vi "Pressure Monitor GUI.vi"(9 "Standalone":bool=TRUE, 10 "Init Data":variant, 11 "My Name":string) -> ()   [LabVIEW 2024]
uses:
  typedefs/CC enum Operation Mode.ctl
  Subsystems/SS typedef cluster Instrument Command Queue Data.ctl
  Subsystems/SS cluster Data Queue type.ctl
  hk-channel-class/hk-channel-class/HK Item/HK Item.lvclass
  CryoCooler/Cryo Cooler/CryoCoolerAVC/CryoCoolerAVC Command cluster.ctl
  CryoCooler/Cryo Cooler/CryoCoolerAVC/CryoCoolerAVC Command enum.ctl
  Pressure Monitor/Pressure Monitor.lvclass
  typedefs/CC cluster Alarm Data.ctl
  Pressure Monitor/CC cluster Pressure Monitor Settings.ctl
  Pressure Monitor/Lesker Pressure/Lesker Pressure.lvclass
  Pressure Monitor/MKS/MKS.lvclass
  hk-channel-class/hk-channel-class/HK Item/HK Item.lvclass/HK Item.ctl
  hk-channel-class/hk-channel-class/HK Item/HK Channel cluster Telemetry Data.ctl
  hk-channel-class/hk-channel-class/HK Item/HK Channel enum Data Type.ctl
  <vilib>/Utility/error.llb/DialogType.ctl
  Pressure Monitor/Lesker Pressure/Lesker Pressure.lvclass/Lesker Pressure.ctl
  hk-channel-class/hk-channel-class/HK Item/Write Source.vi
  CryoCooler/Cryo Cooler/CryoCoolerAVC/CryoCoolerAVC.lvclass
panel:
  in  "Mode":T1
  in  "Tab Control":enum32{"Pressure Monitor", "Engineering", "Log"}(tab)
  in  "Reconnect":bool
  in  "Clear History":bool
  in  "Log Scale":bool=TRUE
  out "Alarm Message":string
  out "Pressure Connected":bool
  out "Alarm":bool
  in  "Status":i32[](listbox) caption="Pressure Monitor"
  out "XY Graph":T2(graph)
  in  "Lesker Notes":string="Guage type is 392\nIf the Ion Gauge commands to turn the filament ON and OFF returns a SYNTAX Error, then you\nneed to go to the gauge front panel menu and select:\nFirst TURN IG OFF, then\nSETUP UNIT > IG CNTL > Set to RS485\n\nSee page 30 of the manual"
  in  "Inst Filament":bool caption="Filament"
  in  "Pump Filament":bool
  in  "Pressure Alarm Level":dbl format="%^_3g"
  in  "Enable Pump Reading?":bool
  in  "Pump Addr":refnum<visa-resource-name>
  in  "Instrument Addr":refnum<visa-resource-name>
  in  "Pressure Type":u16(ring) items=["Simulation", "Lesker", "MKS"]
  in  "Close":bool
  out "Log":string
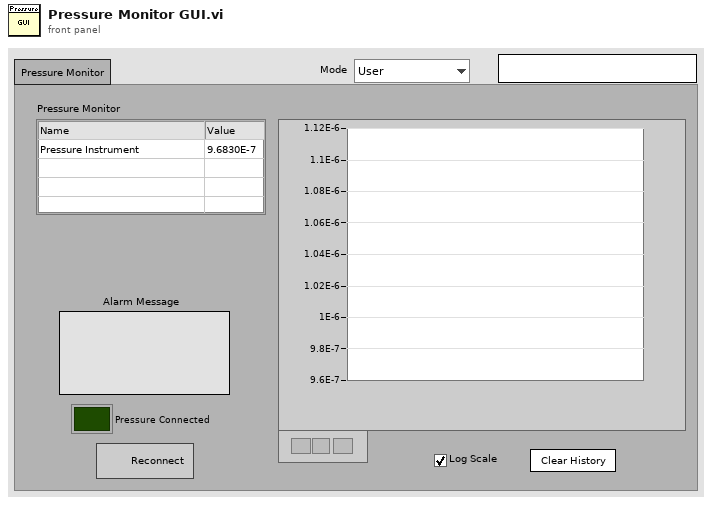
[diagram p1: front panel]
types:
  T1 = typedef "CC enum Operation Mode.ctl" = enum16{"User", "Engineering"}
  T2 = cluster{cluster{"Time Stamp":timestamp, "Numeric":dbl}[]}[]
  T3 = typedef "SS typedef cluster Instrument Command Queue Data.ctl" = cluster{"Cmd":string, "Parameters":variant}
  T4 = typedef "CryoCoolerAVC.lvclass/CryoCoolerAVC Command cluster.ctl" = cluster{"Command":T5, "Options":string, "Cryo Idx":i32}
  T5 = typedef "CryoCoolerAVC.lvclass/CryoCoolerAVC Command enum.ctl" = u16
  T6 = typedef "CC cluster Alarm Data.ctl" = cluster{"Measured Value":dbl, "Alarm Low":dbl, "Alarm High":dbl, "Message":string, "Source":string}
  T7 = typedef "CC cluster Pressure Monitor Settings.ctl" = cluster{"Lesker Addrs":refnum<visa-resource-name>[], "Enabled?":bool[], "Pressure Alarm Level":dbl, "Filaments":bool[]}
  T8 = cluster{"state":refnum<user-event>, "cmd q":refnum<queue>, "Cmd":T3, "Data Q":refnum<queue>, "error":errorcluster, "next poll":timestamp, "My Name":string, "poll":bool, "Channel List":refnum<class "HK Item.lvclass">[], "Focus Pos":dbl, "Data":dbl[], "Cryo Cmd":T4, "Alarm":bool, "PM Ref":refnum<class "Pressure Monitor.lvclass">, "Alarms":T6[], "Source":string, "Settings":T7}
  T9 = typedef "SS cluster Data Queue type.ctl" = cluster{"Source":string, "Type":string, "Data":variant}
  T10 = typedef "HK Item.lvclass/HK Channel enum Data Type.ctl" = enum16{"Floating Point", "Integer", "Enum", "String", "Waveform", "File"}
  T11 = typedef "HK Item.lvclass/HK Channel cluster Telemetry Data.ctl" = cluster{"Ch Names":string[], "Ch Values":dbl[], "Timestamp":timestamp, "Data Type":T10}
  T12 = typedef "CC cluster Device Index.ctl" = cluster{"Device Type Name":string, "Curr Device Name":string, "All Instances":string[]}
  T13 = cluster{"Select Ch":i32[], "Default Device":string}
  T14 = typedef "HK Item.lvclass/HK Channel Units and Setup.ctl" = cluster{"Unit Type":string, "Units":string, "Configuration":string, "Digits":i32, "Data Type":T10, "Exponential?":bool, "Source":string}
  T15 = cluster{cluster{"Time Stamp":timestamp, "Numeric":dbl}[]}
  T16 = typedef "DialogType.ctl" = u16
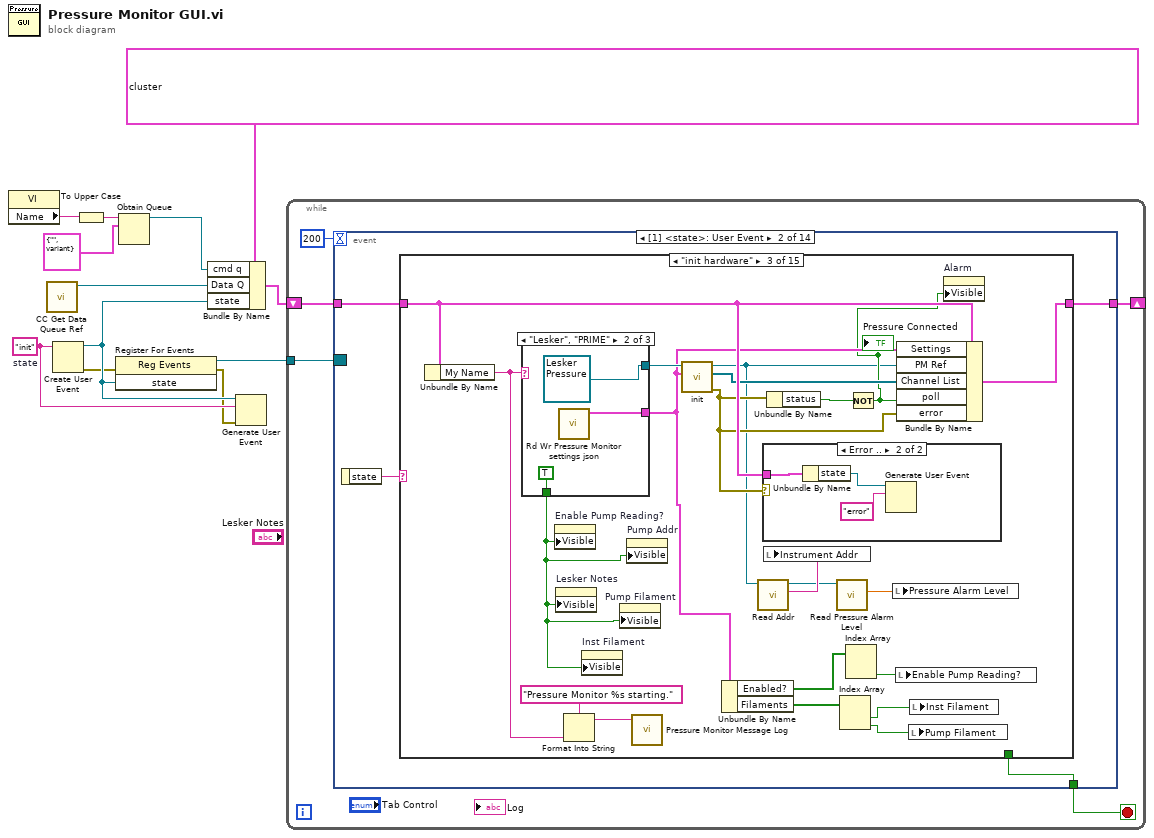
[diagram p0: block diagram]
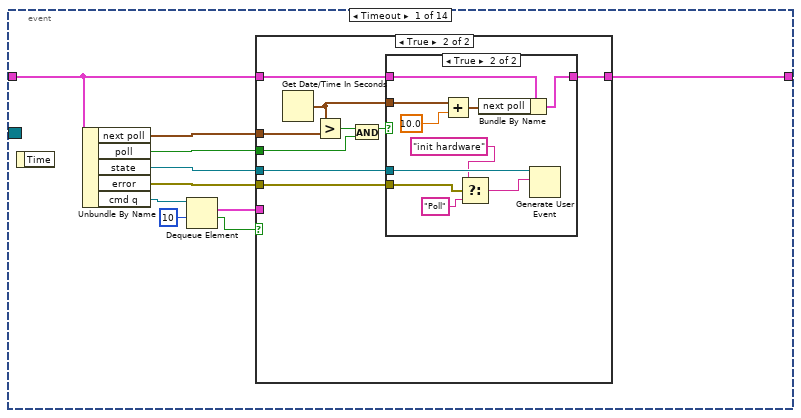
[diagram p2: hidden frame]
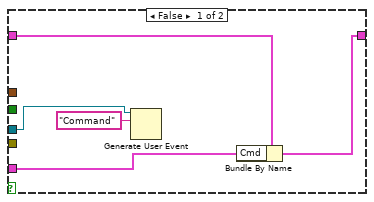
[diagram p3: hidden frame]
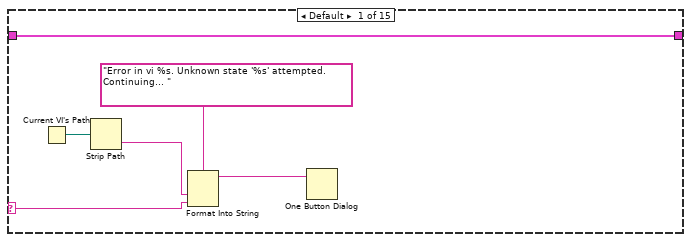
[diagram p5: hidden frame]
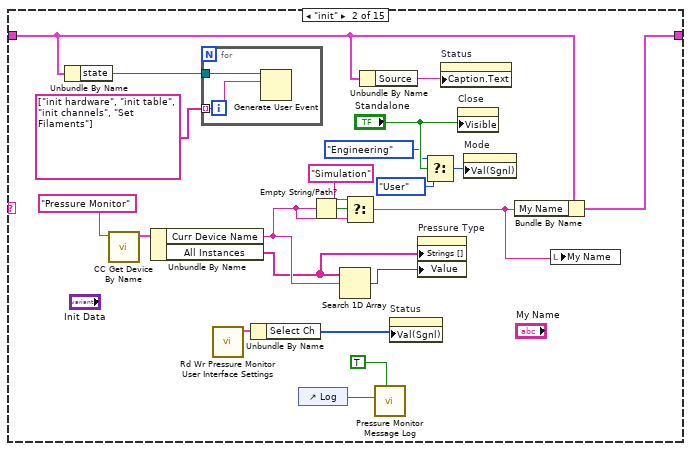
[diagram p6: hidden frame]
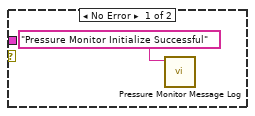
[diagram p7: hidden frame]
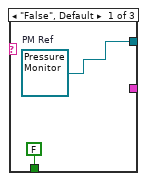
[diagram p8: hidden frame]
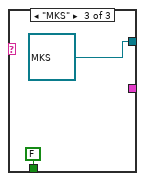
[diagram p9: hidden frame]
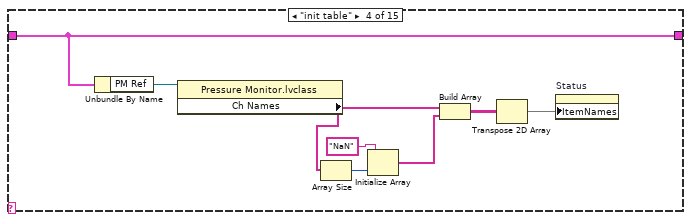
[diagram p10: hidden frame]
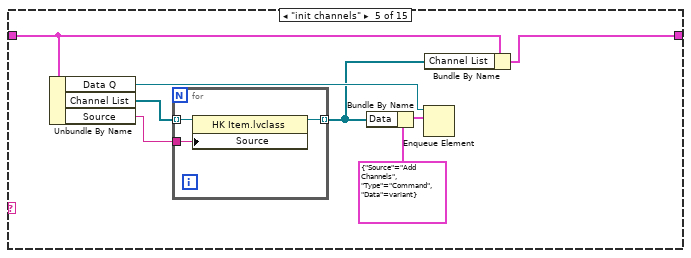
[diagram p11: hidden frame]
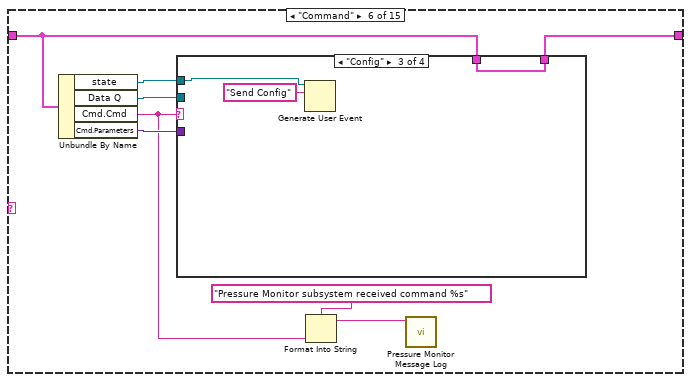
[diagram p12: hidden frame]
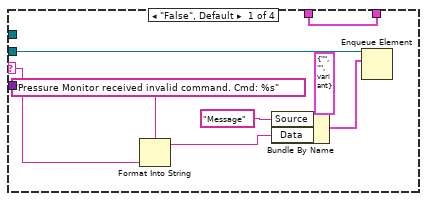
[diagram p13: hidden frame]
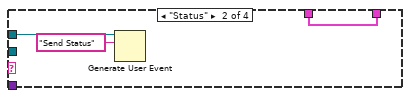
[diagram p14: hidden frame]
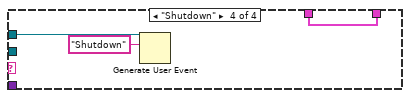
[diagram p15: hidden frame]
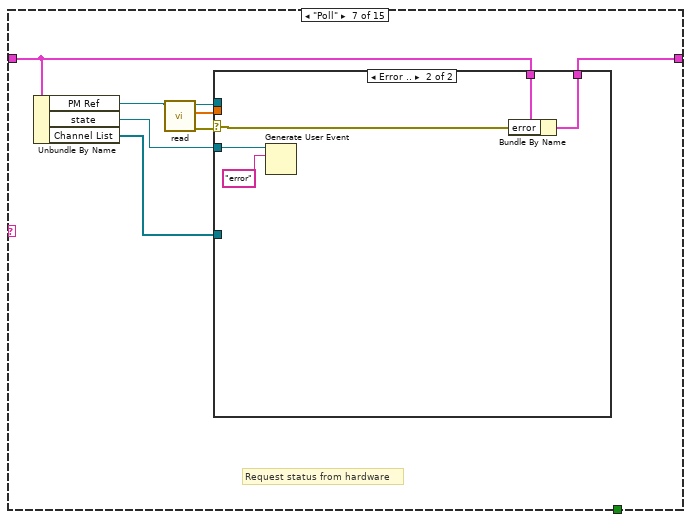
[diagram p16: hidden frame]
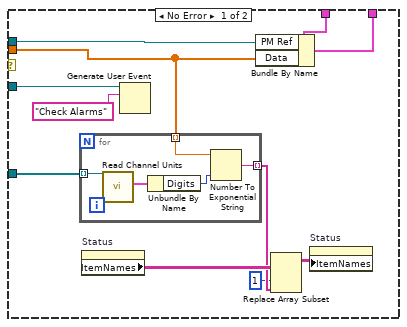
[diagram p17: hidden frame]
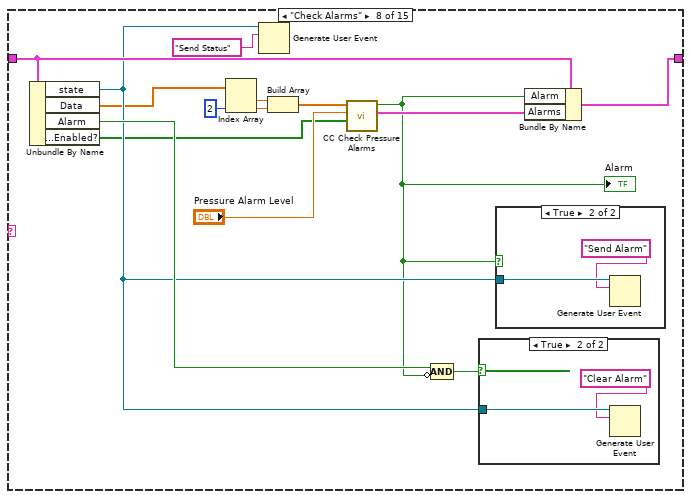
[diagram p18: hidden frame]
diagram:
  w8 = "init"  # state
  n1 = property class="VI"() -> ("Name"=w4:string)  [unwired: 2 in, 2 out]
  n2 = call "CC Get Data Queue Ref.vi"() -> ("Data Q"=w5:refnum<queue>)  [unwired: 10 in, 1 out]
  n3 = Create User Event(user event datatype=w8) -> (user event=w10:refnum<user-event>, error out=w6:errorcluster)  [unwired: 1 in]
  n4 = To Upper Case(1:w4) -> (0:w3:string)
  n5 = register-events(error in=w6, w10) -> (reference out=w9:refnum<event-registration>, error out=w7:errorcluster)  [unwired: 1 in]
  n6 = Obtain Queue(name (unnamed)=w3, element data type=T3 {"Cmd"="", "Parameters"=variant}) -> (queue out=w1:refnum<queue>)  [unwired: 3 in, 2 out]
  n7 = Bundle By Name(cluster=T8 {"state"=refnum, "cmd q"=refnum, "Cmd"={"Cmd"="", "Parameters"=variant}, "Data Q"=refnum, "error"={"status"=FALSE, "code"=0, "source"=""}, "next poll"=timestamp(0 s since 1904-01-01), "My Name"="", "poll"=FALSE, "Channel List"=[], "Focus Pos"=0.0, "Data"=[], "Cryo Cmd"={"Command"=0, "Options"="", "Cryo Idx"=0}, "Alarm"=FALSE, "PM Ref"=refnum, "Alarms"=[], "Source"="Pressure Monitor", "Settings"={"Lesker Addrs"=[], "Enabled?"=[], "Pressure Alarm Level"=0.0001, "Filaments"=[]}}, "cmd q"=w1, "Data Q"=w5, "state"=w10) -> (w11:T8)
  n8 = Generate User Event(user event=w10, event data cluster=w8, error in=w7) -> ()  [unwired: 1 in, 2 out]
  n9 = while {
    tunnel: w9 -> [w17]
    shift-right: [w15] -> _
    shift-left: w11 -> [w16]
    stop <- w14 stop-if-true
    n10 = event shown="[1] <state>: User Event" {
      selector: w17 -> [_ _ _ _ _ _ _ _ _ _ _ _ _ _]
      dyn-events: _ -> [_ _ _ _ _ _ _ _ _ _ _ _ _ _]
      timeout: 200 -> [_ _ _ _ _ _ _ _ _ _ _ _ _ _]
      tunnel: w16 -> [w22 w55 w297 w300 w307 w310 w315 w317 w345 w357 w371 w376 w382 w385]
      tunnel: [w21 w54 w297 w301 w307 w310 w315 w318 w345 w358 w371 w376 w382 w385] -> w15
      tunnel: [_ w53 _ _ _ _ _ _ _ _ _ _ _ _] -> w14
      event Timeout {
        n11 = event-data() -> ()  [unwired: 1 in, 1 out]
        n12 = Unbundle By Name(w22) -> ("next poll"=w20:timestamp, "poll"=w19:bool, "state"=w23:refnum<user-event>, "error"=w18:errorcluster, "cmd q"=w27:refnum<queue>)
        n13 = Dequeue Element(queue=w27, timeout in ms (-1)=10) -> (element=w24:T3, timed out?=w25:bool)  [unwired: 1 in, 2 out]
        n14 = case shown="True" w25 {
          tunnel: w24 -> [w29 _]
          tunnel: w23 -> [w32 w38]
          tunnel: w22 -> [w30 w39]
          tunnel: [w28 w36] -> w21
          tunnel: w20 -> [_ w41]
          tunnel: w19 -> [_ w34]
          tunnel: w18 -> [_ w33]
          frame False {
            n15 = Generate User Event(user event=w32, event data cluster="Command" ("event data")) -> ()  [unwired: 2 in, 2 out]
            n16 = Bundle By Name(cluster=w30, "Cmd"=w29) -> (w28:T8)
          }
          frame True {
            n17 = Get Date/Time In Seconds() -> (seconds since 1Jan1904=w37:timestamp)
            n18 = Greater?(x=w37, y=w41) -> (0:w40:bool)
            n19 = And(x=w40, y=w34) -> (x .and. y?=w35:bool)
            n20 = case shown="True" w35 {
              tunnel: w39 -> [w42 w52]
              tunnel: w38 -> [_ w51]
              tunnel: w37 -> [_ w50]
              tunnel: [w42 w47] -> w36
              tunnel: w33 -> [_ w45]
              frame False {
              }
              frame True {
                n21 = Add(x=w50, y=10.0) -> (x+y=w48:timestamp)
                n22 = Select(t="init hardware" ("event data"), s=w45, f="Poll" ("event data")) -> (s? t:f=w43:string)
                n23 = Bundle By Name(cluster=w52, "next poll"=w48) -> (w47:T8)
                n24 = Generate User Event(user event=w51, event data cluster=w43) -> ()  [unwired: 2 in, 2 out]
              }
            }
          }
        }
      }
      event User Event {
        n25 = event-data() -> ("state"=w56:string)  [unwired: 1 in]
        n26 = case shown="\"init hardware\"" w56 {
          selector: w56 -> [w61 _ _ _ _ _ _ _ _ _ _ _ _ _ _]
          tunnel: w55 -> [w57 w64 w103 w125 w126 w140 w168 w203 w222 w230 w247 w252 w263 w269 w293]
          tunnel: [w57 w82 w106 w125 w127 w141 w169 w204 w222 w230 w247 w253 w264 w270 w293] -> w54
          tunnel: [_ _ _ _ _ _ _ _ _ _ _ _ _ _ TRUE] -> w53
          frame Default {
            n27 = Current VI's Path() -> (path=w60:path)
            n28 = Strip Path(path=w60) -> (name=w59:string)  [unwired: 1 out]
            n29 = Format Into String(format string="Error in vi %s. Unknown state '%s' attempted. Continuing... ", w59, w61) -> (resulting string=w58:string)  [unwired: 2 in, 1 out]
            n30 = One Button Dialog(message=w58) -> ()  [unwired: 1 in, 1 out]
          }
          frame "init" {
            n31 = Unbundle By Name(w64) -> ("state"=w81:refnum<user-event>)
            n32 = call "CC Get Device By Name.vi"("Device Type"="Pressure Monitor") -> ("Device"=w76:T12)  [unwired: 8 in, 2 out]
            n33 = Unbundle By Name(w76) -> ("Curr Device Name"=w75:string, "All Instances"=w74:string[])
            n34 = for {
              tunnel: w81 -> [w85]
              tunnel: string[] ["init hardware", "init table", "init channels", "Set Filaments"] -> [w84] mode=indexing
              n35 = Generate User Event(user event=w85, event data cluster=w84) -> ()  [unwired: 2 in, 2 out]
            }
            n36 = call "Rd Wr Pressure Monitor User Interface Settings.vi"() -> ("Settings"=w66:T13)  [unwired: 10 in, 1 out]
            n37 = Unbundle By Name(w66) -> ("Select Ch"=w65:i32[])
            n38 = control-ref of="Log"() -> (w69:refnum<vi>)
            n39 = Empty String/Path?(string/path=w75) -> (empty?=w83:bool)
            n40 = Search 1D Array(1D array=w74, element=w75) -> (index of element=w79:i32)  [unwired: 1 in]
            n41 = Select(t="Simulation", s=w83, f=w75) -> (s? t:f=w67:string)
            n42 = Unbundle By Name(w64) -> ("Source"=w63:string)
            n43 = call "Pressure Monitor Message Log.vi"("init?"=TRUE, "Log Ref"=w69) -> ()  [unwired: 8 in, 2 out]
            n44 = property on="Status" class="MCListbox (strict)"("Val(Sgnl)"=w65) -> ()  [unwired: 2 in, 2 out]
            n45 = property on="Pressure Type" class="Ring (strict)"("Strings []"=w74, "Value"=w79) -> ()  [unwired: 2 in, 2 out]
            n46 = Select(t=CC_enum_Operation_Mode."Engineering" ("Mode"), s="Standalone", f=CC_enum_Operation_Mode."User" ("Mode")) -> (s? t:f=w70:T1)
            n47 = property on="Status" class="MCListbox (strict)"("Caption.Text"=w63) -> ()  [unwired: 2 in, 2 out]
            n48 = property on="Close" class="Bool"("Visible"="Standalone") -> ()  [unwired: 2 in, 2 out]
            n49 = property on="Mode" class="Enum (strict)"("Val(Sgnl)"=w70) -> ()  [unwired: 2 in, 2 out]
            n50 = Bundle By Name(cluster=w64, "My Name"=w67) -> (w82:T8)
            n51 = local write "My Name"(w67) -> ()
          }
          frame "init hardware" {
            n52 = Unbundle By Name(w103) -> ("My Name"=w105:string)
            n53 = case shown="\"Lesker\", \"PRIME\"" w105 {
              tunnel: [w112 refnum<class "Lesker Pressure.lvclass"> refnum ("Lesker Pressure.lvclass") refnum<class "MKS.lvclass"> refnum ("MKS.lvclass")] -> w101
              tunnel: [_ w115 _] -> w96
              tunnel: [FALSE TRUE FALSE] -> w90
              frame "False", Default {
                w112 = refnum<class "Pressure Monitor.lvclass"> refnum  # PM Ref
              }
              frame "Lesker", "PRIME" {
                n54 = call "Rd Wr Pressure Monitor settings json.vi"() -> ("Pressur Monitor Settings"=w115:T7)  [unwired: 10 in, 1 out]
              }
              frame "MKS" {
              }
            }
            n55 = property on="Enable Pump Reading?" class="Bool (strict)"("Visible"=w90) -> ()  [unwired: 2 in, 2 out]
            n56 = property on="Lesker Notes" class="Str"("Visible"=w90) -> ()  [unwired: 2 in, 2 out]
            n57 = Format Into String(format string="Pressure Monitor %s starting.", w105) -> (resulting string=w102:string)  [unwired: 2 in, 1 out]
            n58 = property on="Inst Filament" class="Bool (strict)"("Visible"=w90) -> ()  [unwired: 2 in, 2 out]
            n59 = property on="Pump Filament" class="Bool (strict)"("Visible"=w90) -> ()  [unwired: 2 in, 2 out]
            n60 = property on="Pump Addr" class="VISAName"("Visible"=w90) -> ()  [unwired: 2 in, 2 out]
            n61 = call "Pressure Monitor Message Log.vi"("String in"=w102) -> ()  [unwired: 9 in, 2 out]
            n62 = call-dynamic "init.vi"("Init Data"=w96, "Pressure Monitor in"=w101) -> ("error out"=w99:errorcluster, "Channel List"=w100:refnum<class "HK Item.lvclass">[], "Pressure Monitor out"=w89:refnum<class "Pressure Monitor.lvclass">)  [unwired: 7 in]
            n63 = Unbundle By Name(w96) -> ("Enabled?"=w98:bool[], "Filaments"=w95:bool[])
            n64 = call-dynamic "Read Addr.vi"("Pressure Monitor in"=w89) -> ("Addr"=w88:string, "Pressure Monitor out"=w87:refnum<class "Pressure Monitor.lvclass">)  [unwired: 8 in, 1 out]
            n65 = case shown="Error .." w99 {
              tunnel: w103 -> [_ w110]
              frame No Error {
                n66 = call "Pressure Monitor Message Log.vi"("String in"="Pressure Monitor Initialize Successful") -> ()  [unwired: 9 in, 2 out]
              }
              frame Error {
                n67 = Unbundle By Name(w110) -> ("state"=w109:refnum<user-event>)
                n68 = Generate User Event(user event=w109, event data cluster="error" ("event data")) -> ()  [unwired: 2 in, 2 out]
              }
            }
            n69 = local write "Instrument Addr"(w88) -> ()
            n70 = Unbundle By Name(w99) -> ("status"=w92:bool)
            n71 = call-dynamic "Read Pressure Alarm Level.vi"("Pressure Monitor in"=w87) -> ("Pressure Alarm Level"=w86:dbl)  [unwired: 8 in, 2 out]
            n72 = Index Array(array=w95) -> (element #1=w94:bool, element #2=w93:bool)  [unwired: 2 in]
            n73 = Index Array(array=w98) -> (element #2=w97:bool)  [unwired: 2 in, 1 out]
            n74 = Not(x=w92) -> (.not. x?=w91:bool)
            "Pressure Connected" <- w91
            n75 = local write "Pressure Alarm Level"(w86) -> ()
            n76 = local write "Enable Pump Reading?"(w97) -> ()
            n77 = Bundle By Name(cluster=w103, "Settings"=w96, "PM Ref"=w89, "Channel List"=w100, "poll"=w91, "error"=w99) -> (w106:T8)
            n78 = local write "Pump Filament"(w93) -> ()
            n79 = local write "Inst Filament"(w94) -> ()
            n80 = property on="Alarm" class="Bool (strict)"("Visible"=w91) -> ()  [unwired: 2 in, 2 out]
          }
          frame "init table" {
            n81 = Unbundle By Name(w125) -> ("PM Ref"=w124:refnum<class "Pressure Monitor.lvclass">)
            n82 = property class="Pressure Monitor.lvclass"(reference=w124) -> ("Ch Names"=w121:string[])  [unwired: 1 in, 2 out]
            n83 = Array Size(array=w121) -> (size(s)=w123:i32)
            n84 = Initialize Array("NaN", w123) -> (w122:string[])
            n85 = Build Array(w121, w122) -> (w119:string[][])
            n86 = Transpose 2D Array(2D array=w119) -> (transposed array=w118:string[][])
            n87 = property on="Status" class="MCListbox (strict)"("ItemNames"=w118) -> ()  [unwired: 2 in, 2 out]
          }
          frame "init channels" {
            n88 = Unbundle By Name(w126) -> ("Data Q"=w131:refnum<queue>, "Channel List"=w130:refnum<class "HK Item.lvclass">[], "Source"=w129:string)
            n89 = for {
              tunnel: w130 -> [w136] mode=indexing
              tunnel: [w135] -> w128 mode=indexing
              tunnel: w129 -> [w134]
              n90 = property class="HK Item.lvclass"(reference=w136, "Source"=w134) -> (reference out=w135:refnum<class "HK Item.lvclass">)  [unwired: 1 in, 1 out]
            }
            n91 = Bundle By Name(cluster=T9 {"Source"="Add Channels", "Type"="Command", "Data"=variant} ("element"), "Data"=w128) -> (w133:T9)
            n92 = Enqueue Element(queue=w131, element=w133) -> ()  [unwired: 2 in, 3 out]
            n93 = Bundle By Name(cluster=w126, "Channel List"=w128) -> (w127:T8)
          }
          frame "Command" {
            n94 = Unbundle By Name(w140) -> ("state"=w142:refnum<user-event>, "Data Q"=w144:refnum<queue>, "Cmd.Cmd"=w138:string, "Cmd.Parameters"=w143:variant)
            n95 = case shown="\"Config\"" w138 {
              selector: w138 -> [w146 _ _ _]
              tunnel: w144 -> [w152 _ _ _]
              tunnel: w143 -> [_ _ _ _]
              tunnel: w142 -> [_ w155 w157 w161]
              tunnel: w140 -> [w145 w153 w156 w159]
              tunnel: [w145 w153 w156 w159] -> w141
              frame "False", Default {
                n96 = Format Into String(format string="Pressure Monitor received invalid command. Cmd: %s", w146) -> (resulting string=w148:string)  [unwired: 2 in, 1 out]
                n97 = Bundle By Name(cluster=T9 {"Source"="", "Type"="", "Data"=variant} ("element"), "Source"="Message" ("Data Type"), "Data"=w148) -> (w147:T9)
                n98 = Enqueue Element(queue=w152, element=w147) -> ()  [unwired: 2 in, 3 out]
              }
              frame "Status" {
                n99 = Generate User Event(user event=w155, event data cluster="Send Status" ("event data")) -> ()  [unwired: 2 in, 2 out]
              }
              frame "Config" {
                n100 = Generate User Event(user event=w157, event data cluster="Send Config" ("event data")) -> ()  [unwired: 2 in, 2 out]
              }
              frame "Shutdown" {
                n101 = Generate User Event(user event=w161, event data cluster="Shutdown" ("event data")) -> ()  [unwired: 2 in, 2 out]
              }
            }
            n102 = Format Into String(format string="Pressure Monitor subsystem received command %s", w138) -> (resulting string=w137:string)  [unwired: 2 in, 1 out]
            n103 = call "Pressure Monitor Message Log.vi"("String in"=w137) -> ()  [unwired: 9 in, 2 out]
          }
          frame "Poll" {
            # "Request status from hardware"
            n104 = Unbundle By Name(w168) -> ("PM Ref"=w165:refnum<class "Pressure Monitor.lvclass">, "state"=w167:refnum<user-event>, "Channel List"=w166:refnum<class "HK Item.lvclass">[])
            n105 = call-dynamic "read.vi"("Pressure Monitor in"=w165) -> ("error out"=w162:errorcluster, "Data"=w163:dbl[], "Pressure Monitor out"=w164:refnum<class "Pressure Monitor.lvclass">)  [unwired: 8 in]
            n106 = case shown="Error .." w162 {
              selector: w162 -> [_ w187]
              tunnel: [w180 w186] -> w169
              tunnel: w168 -> [w179 w188]
              tunnel: w167 -> [w178 w190]
              tunnel: w164 -> [w176 _]
              tunnel: w166 -> [w175 _]
              tunnel: w163 -> [w174 _]
              frame No Error {
                n107 = for {
                  tunnel: w175 -> [w185] mode=indexing
                  tunnel: w174 -> [w182] mode=indexing
                  tunnel: [w181] -> w172 mode=indexing
                  n108 = call "Read Channel Units.vi"("HK Item in"=w185) -> ("Channel Setup"=w184:T14)  [unwired: 8 in, 2 out]
                  n109 = Unbundle By Name(w184) -> ("Digits"=w183:i32)
                  n110 = Number To Exponential String(number=w182, precision (6)=w183) -> (E-format string=w181:string)  [unwired: 2 in]
                }
                n111 = property on="Status" class="MCListbox (strict)"() -> ("ItemNames"=w173:string[][])  [unwired: 2 in, 2 out]
                n112 = Generate User Event(user event=w178, event data cluster="Check Alarms" ("event data")) -> ()  [unwired: 2 in, 2 out]
                n113 = Bundle By Name(cluster=w179, "PM Ref"=w176, "Data"=w174) -> (w180:T8)
                n114 = Replace Array Subset(array=w173, new element=w172, index (col)=1 ("disabled index (col)")) -> (w170:string[][])  [unwired: 1 in]
                n115 = property on="Status" class="MCListbox (strict)"("ItemNames"=w170) -> ()  [unwired: 2 in, 2 out]
              }
              frame Error {
                n116 = Generate User Event(user event=w190, event data cluster="error" ("event data")) -> ()  [unwired: 2 in, 2 out]
                n117 = Bundle By Name(cluster=w188, "error"=w187) -> (w186:T8)
              }
            }
          }
          frame "Check Alarms" {
            n118 = Unbundle By Name(w203) -> ("state"=w200:refnum<user-event>, "Data"=w196:dbl[], "Alarm"=w202:bool, "Settings.Enabled?"=w197:bool[])
            n119 = Index Array(array=w196, index #2=2 ("index")) -> (element #1=w193:dbl, element #2=w194:dbl)  [unwired: 1 in]
            n120 = Generate User Event(user event=w200, event data cluster="Send Status" ("event data")) -> ()  [unwired: 2 in, 2 out]
            n121 = Build Array(w193, w194) -> (w192:dbl[])
            n122 = call "CC Check Pressure Alarms.vi"("Enabled?"=w197, "Pressure Alarm Level"="Pressure Alarm Level", "Presssure Data"=w192) -> ("Alarms"=w198:T6[], "Alarm"=w191:bool)  [unwired: 6 in, 1 out]
            "Alarm" <- w191
            n123 = Compound Arithmetic op=AND(w202, invert w191) -> (w201:bool)
            n124 = case shown="True" w201 {
              tunnel: w200 -> [_ w209]
              frame False {
              }
              frame True {
                n125 = Generate User Event(user event=w209, event data cluster="Clear Alarm" ("event data")) -> ()  [unwired: 2 in, 2 out]
              }
            }
            n126 = case shown="True" w191 {
              tunnel: w200 -> [_ w207]
              frame False {
              }
              frame True {
                n127 = Generate User Event(user event=w207, event data cluster="Send Alarm" ("event data")) -> ()  [unwired: 2 in, 2 out]
              }
            }
            n128 = Bundle By Name(cluster=w203, "Alarm"=w191, "Alarms"=w198) -> (w204:T8)
          }
          frame "Send Alarm" {
            n129 = Unbundle By Name(w222) -> ("Data Q"=w221:refnum<queue>, "Source"=w210:string, "Alarms"=w218:T6[])
            n130 = Index Array(array=w218) -> (element=w212:T6)  [unwired: 1 in]
            n131 = Bundle By Name(cluster=w212, "Source"=w210) -> (w211:T6)
            n132 = Unbundle By Name(w211) -> ("Message"=w215:string)
            n133 = Bundle By Name(cluster=T9 {"Source"="", "Type"="", "Data"=variant} ("element"), "Source"=w210, "Type"="Alarm Set", "Data"=w211) -> (w217:T9)
            n134 = disable-structure shown="Disabled" {
              disable-tunnel: w215 -> [w223 _]
              frame Disabled {
                n135 = call "Pressure Monitor Message Log.vi"("String in"=w223) -> ()  [unwired: 9 in, 2 out]
              }
              frame Enabled {
              }
            }
            n136 = Enqueue Element(queue=w221, element=w217) -> ()  [unwired: 2 in, 3 out]
            n137 = Format Date/Time String() -> (date/time string=w213:string)  [unwired: 3 in]
            n138 = Format Into String(format string=" %s", initial string=w213, w215) -> (resulting string=→"Alarm Message":string)  [unwired: 1 in, 1 out]
          }
          frame "Clear Alarm" {
            w225 = "Alarm condition cleared." ("String in")
            n139 = Unbundle By Name(w230) -> ("Data Q"=w229:refnum<queue>, "Source"=w226:string)
            n140 = Bundle By Name(cluster=T9 {"Source"="", "Type"="", "Data"=variant} ("element"), "Source"=w226, "Type"="Alarm Clear") -> (w224:T9)
            n141 = Enqueue Element(queue=w229, element=w224) -> ()  [unwired: 2 in, 3 out]
            n142 = call "Pressure Monitor Message Log.vi"("String in"=w225) -> ()  [unwired: 9 in, 2 out]
            n143 = local write "Alarm Message"(w225) -> ()
          }
          frame "Send Status" {
            n144 = Unbundle By Name(w247) -> ("Data Q"=w246:refnum<queue>, "Source"=w233:string, "PM Ref"=w232:refnum<class "Pressure Monitor.lvclass">, "Data"=w238:dbl[])
            n145 = Get Date/Time In Seconds() -> (seconds since 1Jan1904=w239:timestamp)
            n146 = call-dynamic "Read Ch Names dyn.vi"("Pressure Monitor in"=w232) -> ("Ch Names"=w231:string[])  [unwired: 8 in, 2 out]
            n147 = Bundle(cluster=T11 {"Ch Names"=[], "Ch Values"=[], "Timestamp"=timestamp(0 s since 1904-01-01), "Data Type"=enum."Floating Point"}, "Ch Names"=w231, "Ch Values"=w238, "Timestamp"=w239, "Data Type"=HK_Channel_enum_Data_Type."Floating Point") -> (w241:T11)
            n148 = call "CC Pressure Monitor Data buffer.vi"("Write?"=TRUE, "Data"=w238, "Time Stamp"=w239) -> ("XY Graph"=w235:T2)  [unwired: 7 in, 1 out]
            n149 = for {
              tunnel: "Status" -> [w249] mode=indexing
              tunnel: w235 -> [w250]
              tunnel: [w248] -> w234 mode=indexing
              n150 = Index Array(array=w250, index=w249) -> (element=w248:T15)
            }
            "XY Graph" <- w234
            n151 = Bundle By Name(cluster=T9 {"Source"="", "Type"="", "Data"=variant} ("element"), "Source"=w233, "Type"="Floating Point" ("Data Type"), "Data"=w241) -> (w243:T9)
            n152 = Enqueue Element(queue=w246, element=w243) -> ()  [unwired: 2 in, 3 out]
          }
          frame "Set Filaments" {
            n153 = Unbundle By Name(w252) -> ("PM Ref"=w255:refnum<class "Pressure Monitor.lvclass">, "Settings.Filaments"=w251:bool[])
            n154 = for {
              shift-right: [w258] -> w254
              shift-left: w255 -> [w259]
              tunnel: w251 -> [w257] mode=indexing
              i -> [w256]
              n155 = call-dynamic "Filament Control.vi"("Filament"=w257, "Filament ID"=w256, "Pressure Monitor in"=w259) -> ("Pressure Monitor out"=w258:refnum<class "Pressure Monitor.lvclass">)  [unwired: 7 in, 1 out]
            }
            n156 = Bundle By Name(cluster=w252, "PM Ref"=w254) -> (w253:T8)
          }
          frame "Reinit" {
            n157 = Unbundle By Name(w263) -> ("PM Ref"=w262:refnum<class "Pressure Monitor.lvclass">, "state"=w266:refnum<user-event>)
            n158 = call-dynamic "close.vi"("Pressure Monitor in"=w262) -> ("error out"=w260:errorcluster, "Pressure Monitor out"=w261:refnum<class "Pressure Monitor.lvclass">)  [unwired: 9 in]
            n159 = Generate User Event(user event=w266, event data cluster="init hardware" ("event data")) -> ()  [unwired: 2 in, 2 out]
            n160 = call <vilib>:"Clear Errors.vi"("error in (no error)"=w260) -> ()  [unwired: 5 in, 2 out]
            n161 = Bundle By Name(cluster=w263, "PM Ref"=w261) -> (w264:T8)
          }
          frame "error" {
            w267 = FALSE ("Pressure Connected")
            w274 = T16 0 items=["no dialog", "OK message", "continue or stop message", "OK message + warnings", "continue/stop + warnings"] ("type of dialog (OK msg:1)")
            # "Wait 3 minutes before trying again"
            n162 = Unbundle By Name(w269) -> ("My Name"=w278:string, "error"=w285:errorcluster, "error.code"=w288:i32, "error.source"=w286:string, "Data Q"=w276:refnum<queue>)
            n163 = local write "Pressure Connected"(w267) -> ()
            n164 = property on="Alarm" class="Bool (strict)"("Visible"=w267) -> ()  [unwired: 2 in, 2 out]
            n165 = property on="Reconnect" class="Bool"("Visible"=TRUE) -> ()  [unwired: 2 in, 2 out]
            n166 = call <vilib>:"Simple Error Handler.vi"("type of dialog (OK msg:1)"=w274, "error in (no error)"=w285) -> ("message"=w284:string)  [unwired: 3 in, 4 out]
            n167 = Bundle By Name(cluster=T6 {"Measured Value"=0.0, "Alarm Low"=0.0, "Alarm High"=0.0, "Message"="", "Source"=""} ("element"), "Source"=w278, "Message"="Pressure Monitor Initialization Error. Check Communications port.") -> (w279:T6)
            n168 = Format Into String(format string="Error from Pressure Monitors \"%s\". Error # %d, Error Source: %s, Error message \"%s\"", w278, w288, w286, w284) -> (resulting string=w283:string)  [unwired: 2 in, 1 out]
            n169 = Bundle By Name(cluster=T9 {"Source"="", "Type"="", "Data"=variant} ("element"), "Source"=w278, "Type"="Alarm Set", "Data"=w279) -> (w275:T9)
            n170 = call "Pressure Monitor Message Log.vi"("String in"=w283) -> ()  [unwired: 9 in, 2 out]
            n171 = Get Date/Time In Seconds() -> (seconds since 1Jan1904=w273:timestamp)
            n172 = Add(x=w273, y=180.0) -> (x+y=w271:timestamp)
            n173 = Enqueue Element(queue=w276, element=w275) -> ()  [unwired: 2 in, 3 out]
            n174 = Bundle By Name(cluster=w269, "next poll"=w271) -> (w270:T8)
          }
          frame "Shutdown" {
            n175 = Unbundle By Name(w293) -> ("Data Q"=w292:refnum<queue>, "PM Ref"=w290:refnum<class "Pressure Monitor.lvclass">)
            n176 = Release Queue(queue=w292) -> ()  [unwired: 2 in, 3 out]
            n177 = call-dynamic "close.vi"("Pressure Monitor in"=w290) -> ("error out"=w289:errorcluster)  [unwired: 9 in, 1 out]
            n178 = call "Pressure Monitor Message Log.vi"("String in"="Pressure Monitor shutting down.") -> ()  [unwired: 9 in, 2 out]
            n179 = call <vilib>:"Clear Errors.vi"("error in (no error)"=w289) -> ()  [unwired: 5 in, 2 out]
          }
        }
      }
      event "Reconnect": Value Change {
        n180 = event-data() -> ()  [unwired: 1 in, 6 out]
        n181 = Unbundle By Name(w297) -> ("state"=w296:refnum<user-event>)
        n182 = Generate User Event(user event=w296, event data cluster="init hardware" ("event data")) -> ()  [unwired: 2 in, 2 out]
      }
      event "Pump Filament", "Inst Filament": Value Change {
        n183 = event-data() -> ()  [unwired: 1 in, 6 out]
        n184 = Unbundle By Name(w300) -> ("state"=w299:refnum<user-event>)
        n185 = Generate User Event(user event=w299, event data cluster="Set Filaments" ("event data")) -> ()  [unwired: 2 in, 2 out]
        n186 = Build Array("Inst Filament", "Pump Filament") -> (w302:bool[])
        n187 = Bundle By Name(cluster=w300, "Settings.Filaments"=w302) -> (w301:T8)
      }
      event "Log Scale": Value Change {
        n188 = event-data() -> ()  [unwired: 1 in, 6 out]
        n189 = Boolean To (0,1)(Boolean="Log Scale") -> (0, 1=w305:i16)
        n190 = property on="XY Graph" class="XYGraph (strict)"("YScale.Mapping Mode"=w305) -> ()  [unwired: 2 in, 2 out]
      }
      event "Clear History": Value Change {
        n191 = event-data() -> ()  [unwired: 1 in, 6 out]
        n192 = call "CC Pressure Monitor Data buffer.vi"("Clear"=TRUE, "Write?"=FALSE) -> ()  [unwired: 8 in, 2 out]
      }
      event "Pressure Alarm Level": Value Change {
        n193 = event-data() -> ("NewVal"=w313:dbl)  [unwired: 1 in]
        n194 = call "Rd Wr Pressure Monitor settings json.vi"() -> ("Pressur Monitor Settings"=w314:T7)  [unwired: 10 in, 1 out]
        n195 = Bundle By Name(cluster=w314, "Pressure Alarm Level"=w313) -> (w312:T7)
        n196 = call "Rd Wr Pressure Monitor settings json.vi"("Write? (F:Read)"=TRUE, "Pressur Monitor Settings"=w312) -> ()  [unwired: 8 in, 2 out]
      }
      event "Enable Pump Reading?": Value Change {
        n197 = event-data() -> ()  [unwired: 1 in, 6 out]
        n198 = Unbundle By Name(w317) -> ("My Name"=w316:string, "PM Ref"=w320:refnum<class "Pressure Monitor.lvclass">)
        n199 = case shown="\"PRIME\"" w316 {
          tunnel: w320 -> [_ w335]
          tunnel: "Enable Pump Reading?" -> [_ w330]
          tunnel: [w321 w327] -> w318
          tunnel: w317 -> [w321 w326]
          frame "False", Default {
          }
          frame "PRIME" {
            n200 = To More Specific Class(target class=refnum<class "Lesker Pressure.lvclass"> refnum ("Lesker Pressure.lvclass"), reference=w335) -> (specific class reference=w334:refnum<class "Lesker Pressure.lvclass">)  [unwired: 1 in, 1 out]
            n201 = call "Rd Wr Pressure Monitor settings json.vi"() -> ("Pressur Monitor Settings"=w325:T7)  [unwired: 10 in, 1 out]
            n202 = call "Read Enabled_.vi"("Lesker Pressure in"=w334) -> ("Enabled?"=w332:bool[], "Lesker Pressure out"=w329:refnum<class "Lesker Pressure.lvclass">)  [unwired: 8 in, 1 out]
            n203 = Replace Array Subset(array=w332, new element=w330, index=1) -> (w323:bool[])
            n204 = Bundle By Name(cluster=w325, "Enabled?"=w323) -> (w322:T7)
            n205 = call "Write Enabled_.vi"("Enabled?"=w323, "Lesker Pressure in"=w329) -> ("Lesker Pressure out"=w328:refnum<class "Lesker Pressure.lvclass">)  [unwired: 8 in, 1 out]
            n206 = Bundle By Name(cluster=w326, "PM Ref"=w328, "Settings"=w322) -> (w327:T8)
            n207 = call "Rd Wr Pressure Monitor settings json.vi"("Write? (F:Read)"=TRUE, "Pressur Monitor Settings"=w322) -> ()  [unwired: 8 in, 2 out]
          }
        }
      }
      event "Status": Value Change {
        n208 = event-data() -> ("NewVal"=w340:i32[])  [unwired: 1 in]
        n209 = call "CC Pressure Monitor Data buffer.vi"() -> ("XY Graph"=w344:T2)  [unwired: 10 in, 1 out]
        n210 = call "Rd Wr Pressure Monitor User Interface Settings.vi"() -> ("Settings"=w341:T13)  [unwired: 10 in, 1 out]
        n211 = for {
          tunnel: w340 -> [w347] mode=indexing
          tunnel: w344 -> [w348]
          tunnel: [w346] -> w343 mode=indexing
          n212 = Index Array(array=w348, index=w347) -> (element=w346:T15)
        }
        n213 = Bundle By Name(cluster=w341, "Select Ch"=w340) -> (w339:T13)
        n214 = Unbundle By Name(w345) -> ("PM Ref"=w337:refnum<class "Pressure Monitor.lvclass">)
        n215 = call-dynamic "Read Ch Names dyn.vi"("Pressure Monitor in"=w337) -> ("Ch Names"=w336:string[])  [unwired: 8 in, 2 out]
        n216 = call "Rd Wr Pressure Monitor User Interface Settings.vi"("Write? (F:Read)"=TRUE, "Settings"=w339) -> ()  [unwired: 8 in, 2 out]
        n217 = property on="XY Graph" class="XYGraph (strict)"("Value"=w343) -> (error out=w342:errorcluster)  [unwired: 2 in, 1 out]
        n218 = for {
          N -> [w350]
          tunnel: w340 -> [w353] mode=indexing
          tunnel: w336 -> [w354]
          tunnel: w342 -> [w349]
          i -> [w352]
          n219 = Index Array(array=w354, index=w353) -> (element=w351:string)
          n220 = property on="XY Graph" class="XYGraph (strict)"(error in=w349, "Active Plot"=w352, "Plot.Plot Name"=w351, "LegNumRows"=w350) -> ()  [unwired: 1 in, 2 out]
        }
      }
      event "Pressure Type": Value Change {
        n221 = event-data() -> ("CtlRef"=w362:refnum<vi>)  [unwired: 1 in, 5 out]
        n222 = property class="Ring (strict)"(reference=w362) -> ("Strings []"=w361:string[])  [unwired: 1 in, 2 out]
        n223 = Unbundle By Name(w357) -> ("state"=w356:refnum<user-event>)
        n224 = Generate User Event(user event=w356, event data cluster="Reinit" ("event data")) -> ()  [unwired: 2 in, 2 out]
        n225 = Index Array(array=w361, index="Pressure Type") -> (element=w359:string)
        n226 = Bundle By Name(cluster=w357, "My Name"=w359) -> (w358:T8)
      }
      event "Instrument Addr", "Pump Addr": Value Change {
        n227 = event-data() -> ()  [unwired: 1 in, 6 out]
        n228 = call "Rd Wr Pressure Monitor settings json.vi"("Write? (F:Read)"=FALSE) -> ("Pressur Monitor Settings"=w367:T7)  [unwired: 9 in, 1 out]
        n229 = Unbundle By Name(w371) -> ("state"=w370:refnum<user-event>)
        n230 = Build Array("Instrument Addr", "Pump Addr") -> (w363:refnum<visa-resource-name>[])
        n231 = Generate User Event(user event=w370, event data cluster="Reinit" ("event data")) -> ()  [unwired: 2 in, 2 out]
        n232 = Bundle By Name(cluster=w367, "Lesker Addrs"=w363) -> (w366:T7)
        n233 = call "Rd Wr Pressure Monitor settings json.vi"("Write? (F:Read)"=TRUE, "Pressur Monitor Settings"=w366) -> ()  [unwired: 8 in, 2 out]
      }
      event Value Change {
        n234 = event-data() -> ()  [unwired: 1 in, 6 out]
        n235 = case shown="\"User\", Default" "Mode" {
          tunnel: [bool[] [TRUE, FALSE, FALSE] bool[] [TRUE, TRUE, TRUE]] -> w373
          frame "User", Default {
          }
          frame "Engineering" {
          }
        }
        n236 = property on="Tab Control" class="TabCtl (strict)"() -> ("Pages"=w374:refnum<vi>[])  [unwired: 2 in, 2 out]
        n237 = for {
          tunnel: w374 -> [w378] mode=indexing
          tunnel: w373 -> [w377] mode=indexing
          n238 = property class="Page"(reference=w378, "PageVis"=w377) -> ()  [unwired: 1 in, 2 out]
        }
      }
      event "Standalone": Value Change {
        n239 = event-data() -> ("NewVal"=w381:bool)  [unwired: 1 in, 5 out]
        n240 = property on="Close" class="Bool"("Visible"=w381) -> ()  [unwired: 2 in, 2 out]
      }
      event "Close": Value Change {
        n241 = event-data() -> ()  [unwired: 1 in, 2 out]
        n242 = Unbundle By Name(w385) -> ("state"=w384:refnum<user-event>)
        n243 = Generate User Event(user event=w384, event data cluster="Shutdown" ("event data")) -> ()  [unwired: 2 in, 2 out]
      }
    }
  }
